vi "generateWaveform.vi"(8 "error in (no error)":errorcluster, 11 "SineWave in":refnum<class "SineWave.lvclass">) -> (0 "error out":errorcluster, 2 "Output":dbl, 3 "SineWave out":refnum<class "SineWave.lvclass">)   [LabVIEW 2015, in "SineWave.lvclass"]
uses:
  SineWave.lvclass
  <vilib>/ptbypt/NI_PtbyPt.lvlib
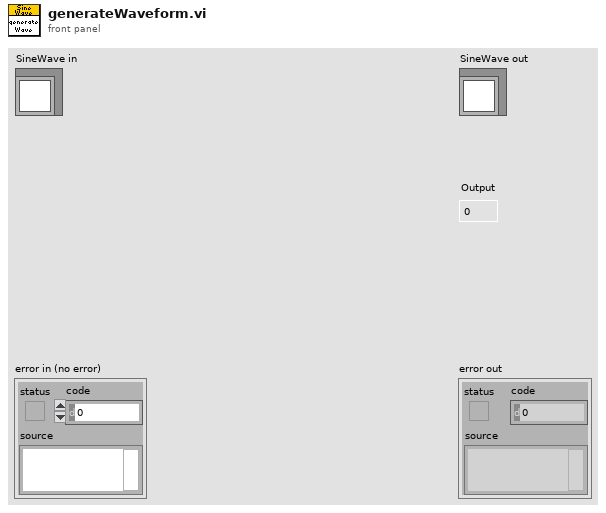
[diagram p1: front panel]
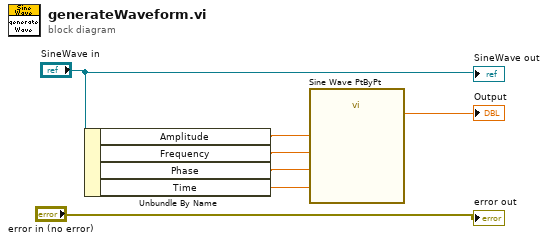
[diagram p0: block diagram]
diagram:
  n1 = Unbundle By Name("SineWave in") -> ("Amplitude"=w5:dbl, "Frequency"=w4:dbl, "Phase"=w3:dbl, "Time"=w2:dbl)
  n2 = call <vilib>:"Sine Wave PtByPt.vi"("time"=w2, "phase"=w3, "frequency"=w4, "amplitude"=w5) -> ("sine wave"=→"Output":dbl)
  "error out" <- "error in (no error)"
  "SineWave out" <- "SineWave in"
